vi "set_position.vi"(10 "position":i32, 11 "Block in":refnum<class "Block.lvclass">) -> (3 "Block out":refnum<class "Block.lvclass">)   [LabVIEW 2020, in "lvdata.lvlib" / "Block.lvclass"]
uses:
  Block.lvclass
  Block.lvclass/Block.ctl
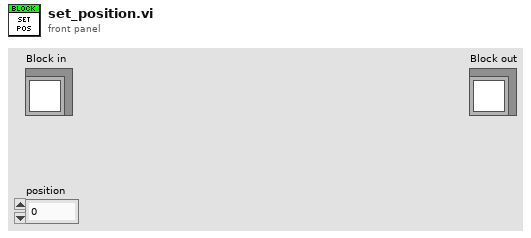
[diagram p1: front panel]
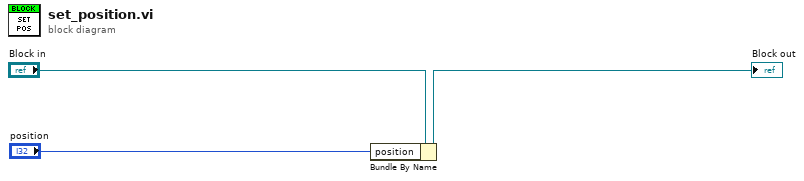
[diagram p0: block diagram]
diagram:
  n1 = Bundle By Name(cluster="Block in", "position"="position") -> (→"Block out":refnum<class "Block.lvclass">)
